vi "SQLite Delete Items of TestSequence.vi"(8 "error in (no error)":errorcluster, 11 "Main":string="0") -> (0 "error out":errorcluster, 5 "Main Out":string)   [LabVIEW 2017, in "SQLite.lvclass"]
doc: "delete items from TestSequence Table.\n2016-09-01 15:46:14\n蒋松\njiangsong@outlook.com"
uses:
  SQLite.lvclass
  SQLiteFileName.ctl
  TabelFullName.ctl
  <userlib>/LabSQL/LabSQL.lvlib
  <userlib>/sushu/sushu.lvlib
panel:
  out "Select SQL CMD":string
  # "sfdgs\nsfdgs"
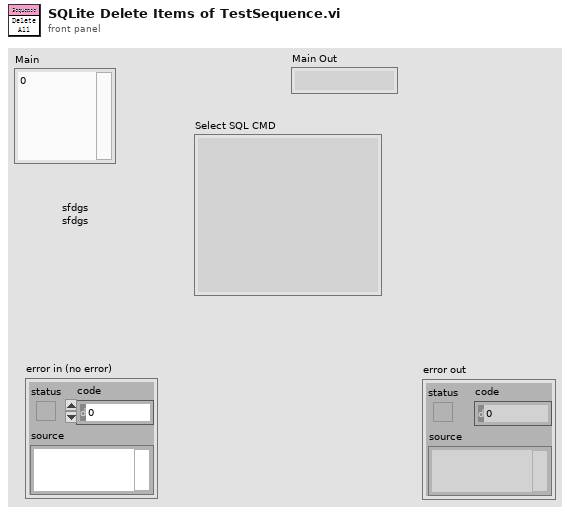
[diagram p1: front panel]
types:
  T1 = typedef "SQLite.lvclass/TabelFullName.ctl" = string
  T2 = typedef "SQLite.lvclass/SQLiteFileName.ctl" = string
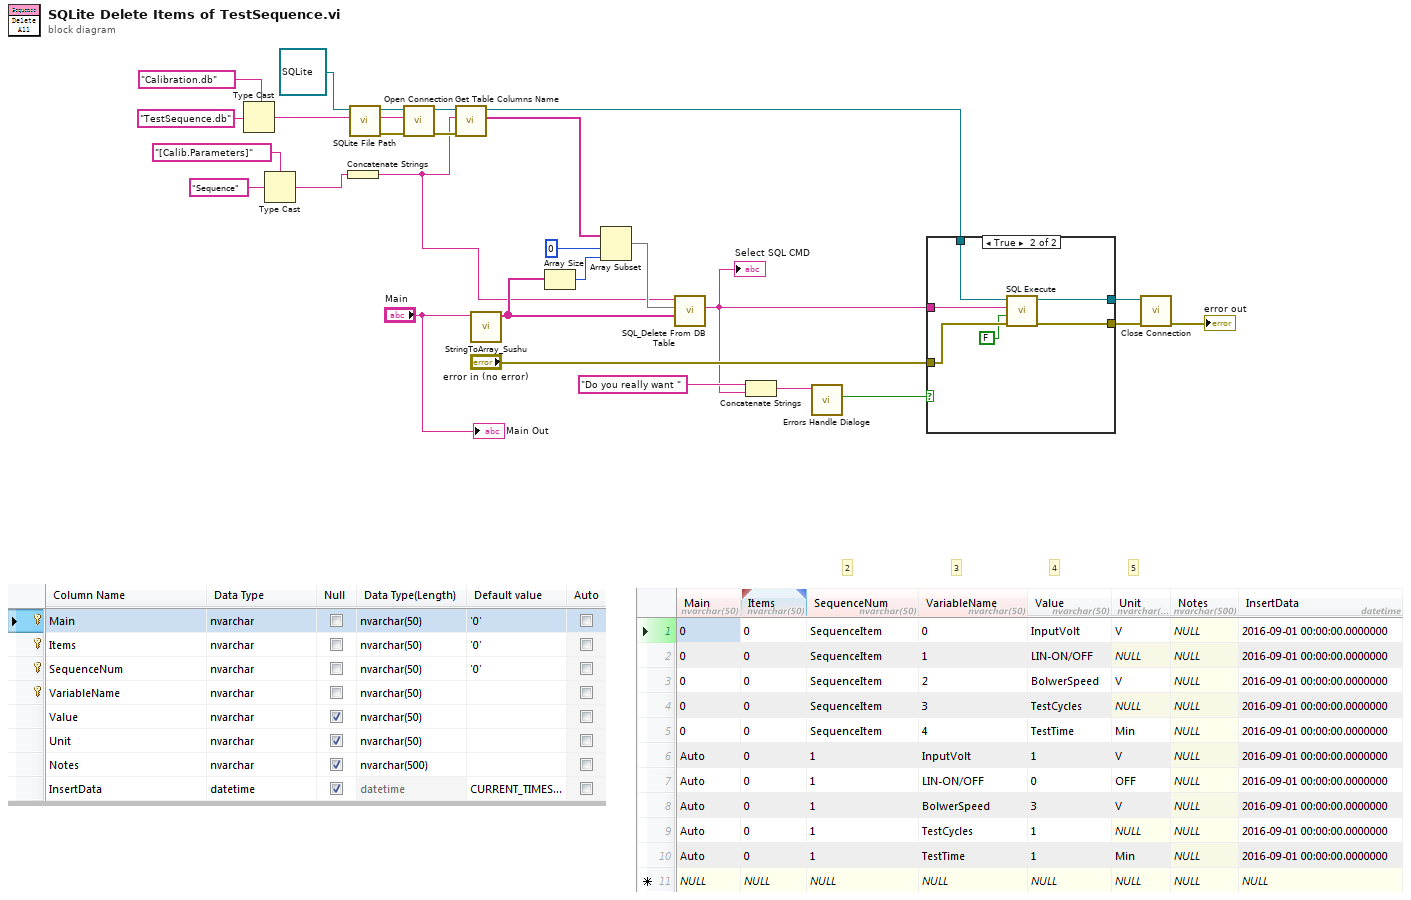
[diagram p0: block diagram]
diagram:
  # "5"
  # "4"
  # "3"
  # "2"
  n1 = Type Cast(type=T2 "Calibration.db" ("SQLiteFileName"), x="TestSequence.db" ("Remaining States")) -> (*(type *) &x=w15:T2)
  n2 = Type Cast(type=T1 "[Calib.Parameters]" ("TabelFullName"), x="Sequence" ("Remaining States")) -> (*(type *) &x=w18:T1)
  n3 = Concatenate Strings(w18) -> (w4:string)
  n4 = call "SQLite File Path.vi"("SQLiteFileName"=w15, "SQLite in"=refnum<class "SQLite.lvclass"> refnum ("SQLite.lvclass")) -> ("error out"=w12:errorcluster, "string"=w9:string, "SQLite out"=w11:refnum<class "SQLite.lvclass">)  [unwired: 7 in]
  n5 = call-dynamic "Open Connection.vi"("error in (no error)"=w12, "ConnectionString"=w9, "HostDB in"=w11) -> ("error out"=w8:errorcluster, "HostDB out"=w7:refnum<class "SQLite.lvclass">)  [unwired: 7 in]
  n6 = call-dynamic "Get Table Columns Name.vi"("error in (no error)"=w8, "TableName"=w4, "HostDB in"=w7) -> ("ColunmsList"=w5:string[], "HostDB out"=w6:refnum<class "SQLite.lvclass">)  [unwired: 4 in, 3 out]
  n7 = call <userlib>:"StringToArray_Sushu.vi"("State Queue"="Main") -> ("Array"=w25:string[])  [unwired: 8 in, 2 out]
  n8 = Array Size(array=w25) -> (size(s)=w26:i32)
  n9 = Array Subset(array=w5, index=0 ("length"), length=w26) -> (w23:string[])
  n10 = call <userlib>:"SQL_Delete From DB Table.vi"("ColumnsValue"=w25, "ColumnsNameList"=w23, "TableName"=w4) -> ("Select SQL CMD"=w21:string)  [unwired: 8 in]
  "Select SQL CMD" <- w21
  n11 = Concatenate Strings("Do you really want " ("string"), w21) -> (w20:string)
  n12 = call <userlib>:"Errors Handle Dialoge.vi"("Message"=w20) -> ("OK?"=w19:bool)  [unwired: 9 in, 1 out]
  n13 = case shown="True" w19 {
    tunnel: "error in (no error)" -> [w29 w33]
    tunnel: w6 -> [w30 w36]
    tunnel: [w30 w35] -> w3
    tunnel: [w29 w32] -> w2
    tunnel: w21 -> [_ w34]
    frame False {
    }
    frame True {
      n14 = call-dynamic "SQL Execute.vi"("error in (no error)"=w33, "Return Data (T)"=FALSE, "Command Text"=w34, "HostDB in"=w36) -> ("error out"=w32:errorcluster, "HostDB out"=w35:refnum<class "SQLite.lvclass">)  [unwired: 3 in, 3 out]
    }
  }
  n15 = call-dynamic "Close Connection.vi"("error in (no error)"=w2, "HostDB in"=w3) -> ("error out"=→"error out":errorcluster)  [unwired: 8 in, 1 out]
  "Main Out" <- "Main"
